vi "国标仪器获取仪器状态.vi"(8 "error in (no error)":errorcluster, 11 "站号":u16(ring)=3 items=["总磷"=1, "总氮"=2, "氨氮"=3, "CODMn"=21, "CODCr"=22]) -> (0 "error out":errorcluster, 3 "状态告警区":T1 {"告警代码" items=["无告警", "缺试剂告警", "缺水样告警", "缺蒸馏水告警", "缺标液告警", "仪表漏液告警", "标定异常告警", "超量程告警", "加热异常", "低试剂预警", "超上限告警", "超下限告警", "仪表内部其他异常", "滴定异常告警", "电极异常告警", "量程切换告警", "参数设置告警", "PH电极电位异常", "电导率电极异常", "浊度光度异常", "溶解氧电极异常", "溶解氧光强异常", "温度异常告警", "PH异常告警", "溶解氧异常告警", "电导率异常告警", "浊度异常告警", "叶绿素异常告警", "藻密度异常告警", "蓝绿藻异常告警", "ORP异常告警", "氨氮异常告警", "清洁刷异常告警", "SD卡异常告警", "蓝牙异常告警", "Wifi异常告警", "流程异常告警"]; "故障代码" items=["无故障", "电机故障", "温度故障", "通讯故障", "滴定故障"]})   [LabVIEW 2016, in "质控单元V2.lvlib"]
uses:
  <vilib>/Plasmionique/MB Master/MB_Master/MB_Master.lvclass
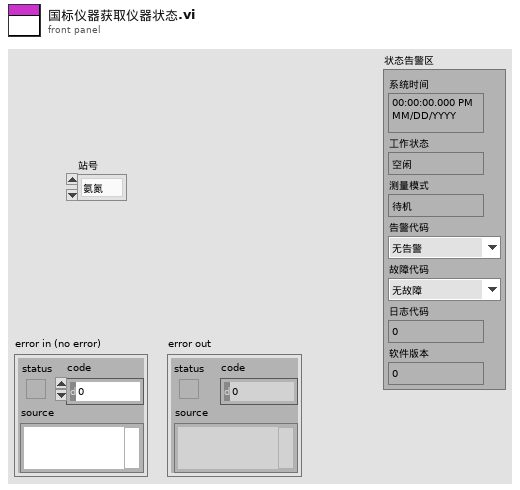
[diagram p1: front panel]
types:
  T1 = cluster{"系统时间":timestamp, "工作状态":enum16{"空闲", "水样测试", "标样核查", "零点核查", "跨度核查", "空白测试", "平行样测试", "加标回收", "空白校准", "标样校准", "初始化（清洗）"}, "测量模式":enum16{"待机", "连续模式", "周期模式", "定点模式", "受控模式", "手动模式"}, "告警代码":u16, "故障代码":u16, "日志代码":u16, "软件版本":u16}
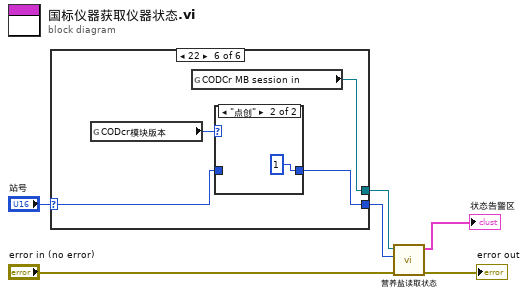
[diagram p0: block diagram]
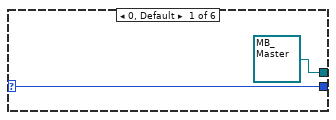
[diagram p2: hidden frame]
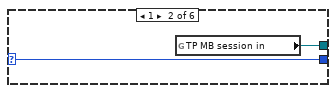
[diagram p3: hidden frame]
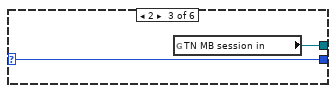
[diagram p4: hidden frame]
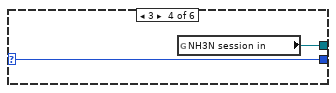
[diagram p5: hidden frame]
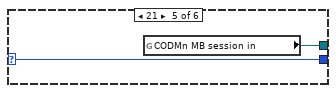
[diagram p6: hidden frame]
diagram:
  n1 = case shown="22" "站号" {
    selector: "站号" -> [w7 w9 w11 w13 w15 w18]
    tunnel: [refnum<class "MB_Master.lvclass"> refnum ("CODMn MB session in") w10 w12 w14 w16 w20] -> w6
    tunnel: [w7 w9 w11 w13 w15 w17] -> w1
    frame 0, Default {
    }
    frame 1 {
      n2 = global read "系统交互.vi" "TP MB session in"() -> (w10:refnum<class "MB_Master.lvclass">)
    }
    frame 2 {
      n3 = global read "系统交互.vi" "TN MB session in"() -> (w12:refnum<class "MB_Master.lvclass">)
    }
    frame 3 {
      n4 = global read "系统交互.vi" "NH3N session in"() -> (w14:refnum<class "MB_Master.lvclass">)
    }
    frame 21 {
      n5 = global read "系统交互.vi" "CODMn MB session in"() -> (w16:refnum<class "MB_Master.lvclass">)
    }
    frame 22 {
      n6 = global read "系统交互.vi" "CODcr模块版本"() -> (w19:enum16{"斯坦道V3", "点创"})
      n7 = global read "系统交互.vi" "CODCr MB session in"() -> (w20:refnum<class "MB_Master.lvclass">)
      n8 = case shown="\"点创\"" w19 {
        tunnel: w18 -> [w21 _]
        tunnel: [w21 u16 1 ("站号")] -> w17
        frame "斯坦道V3", Default {
        }
        frame "点创" {
        }
      }
    }
  }
  n9 = call "营养盐读取状态.vi"("error in (no error)"="error in (no error)", "站号"=w1, "MB session in"=w6) -> ("error out"=→"error out":errorcluster, "状态告警区"=→"状态告警区":T1)  [unwired: 7 in]
